vi "save_batch+info_files.vi.vi"(0 "Current PulseBlaster Array":T5(array[cluster]), 1 "6713 DAC Array":dbl[](array[numeric]), 2 "Save in second location?":bool, 3 "detuning values":T4={"flaser"=-22.0, "fimage"=14.997, "fmot"=-56.5, "fzeeman"=-524.0, "f2dcollimator"=-22.0, "fmolecule"=-2225.6} {"fmolecule" format="%.2f"; "f2dcollimator" format="%.2f"; "fzeeman" format="%.2f"; "fmot" format="%.2f"; "fimage" format="%.2f"; "flaser" format="%.2f"}, 4 "2scope filename":string, 5 "wavemeter reading":string, 6 "Drop Time Column":i32=16, 7 "Parameters to Change":T1={"PB parameter to change"=0, "Column of\nData to Change"=0, "Column of\nDelay to Change"=9, "6713 DAC Ch\nto Change"=7, "column for Wvfrm\n(red mot cooling)"=10, "# of PB arrays"=1, "column for Wvrm\nODT"=10, "TrimCurrent\nCh to Chng"=1} {"TrimCurrent\nCh to Chng" min=1 max=2; "PB parameter to change" min=0 max=4}, 8 "base path":path, 9 "saved image dimensions":i32[](array[numeric]), 10 "Cut Images\nin Software?":bool=TRUE, 11 "Array of monitor outputs":dbl[](array[numeric]), 12 "ROI Parameters":T2={"Col Start"=45, "Col Length"=125, "Row Start"=105, "Row Length"=130}, 13 "Software Binning\n(occurs before saving)":T3={"Software\nBinning?"=TRUE, "Software Bin Size"=4}, 14 "Base File Name":string="redMOTtemp0441" caption="Base File Name (filename, base delay of column 10, and .dat will be added as extension.", 15 "Changed Value":dbl=165.25000000000003, 16 "arbitrary info string":string, 17 "Software\nSumming":u32=10, 18 "alternate path":path, 19 "Analog Input Ch \nto Save to Batch":i32, 20 "Opt trap Wvfrm array":waveform(dbl)[](array[waveform]), 22 "ODT Wvfrm trigger column":i32=16, 23 "PixelFly y bin":i32, 24 "PixelFly x bin":i32, 26 "Opt Trap off column":i32=16, 27 "iteration #":i32) -> (25 "filename component":string)   [LabVIEW 2013]
doc: "This VI concatenates various information of interest to form the file name component that goes before the extension (and possibly another modifier such as \"atoms\" or \"background\")."
uses:
  <vilib>/Waveform/WDTOps.llb/WDT Index Channel DBL.vi
  <vilib>/Waveform/WDTOps.llb/WDT Waveform Duration DBL.vi
  <vilib>/Waveform/WDTOps.llb/WDT Get XY Value DBL.vi
panel:
  in  "BEC Peak weight":i32
  in  "Thermal width guess":i32=10
  in  "BEC width guess":i32=25
  out "6713 dac1 string":string
  out "6713 DAC CH0":string
  out "waveform 2":waveform(dbl)(graph)
  out "waveform":waveform(dbl)(graph)
  out "Dimple value":dbl format="%.3f"
  out "ODT value":dbl format="%.3f"
  in  "Gain (har wired)":i32(ring) items=["Low (X1)", "High (X2)"]
  out "opt trap off time (along wvfrm)":dbl
  in  "Image Beam Column":i32=23
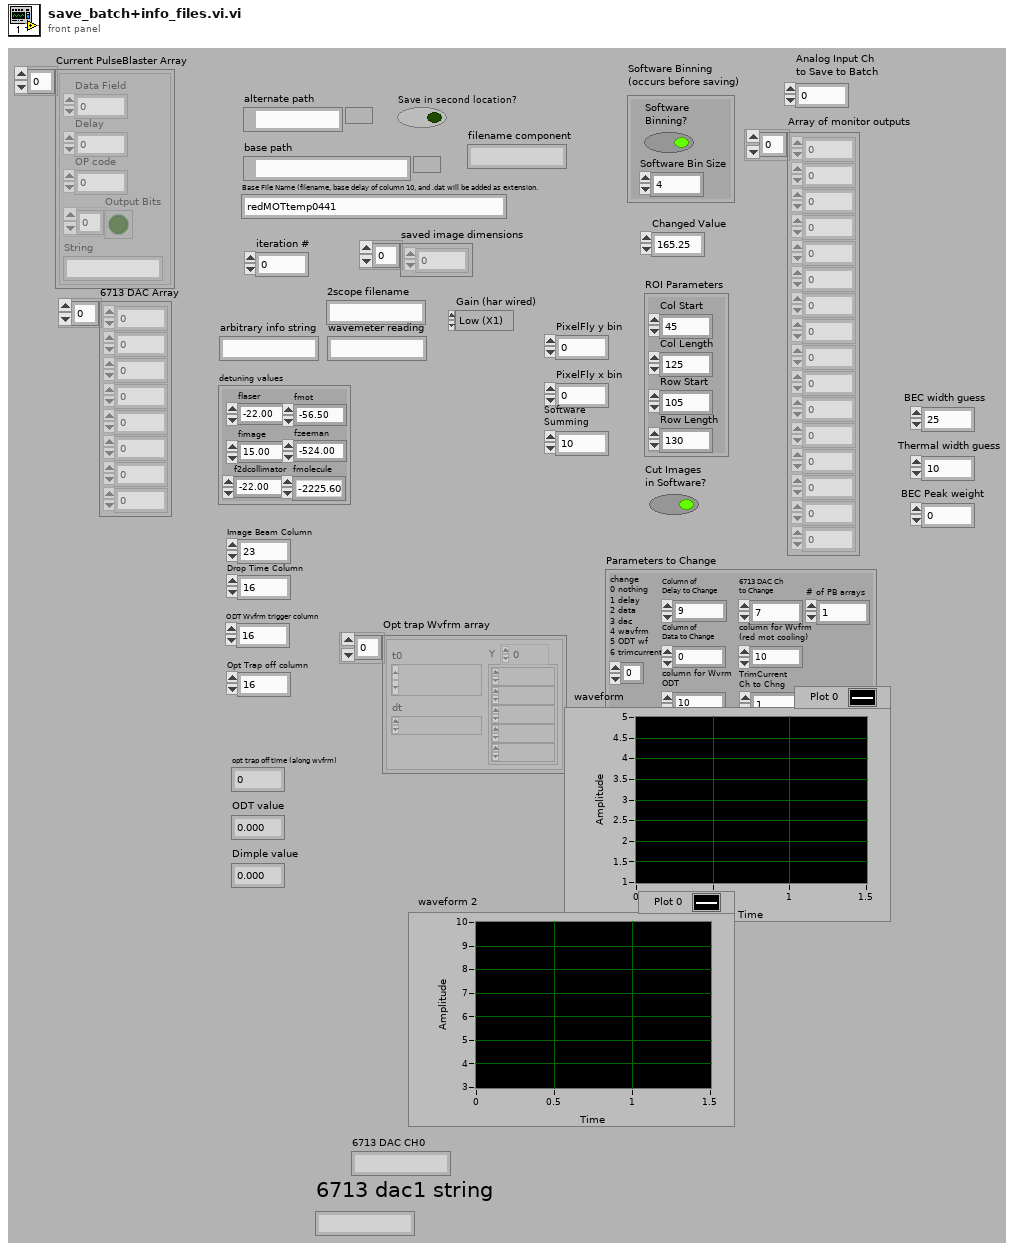
[diagram p1: front panel]
types:
  T1 = cluster{"PB parameter to change":i8, "Column of\nData to Change":i32, "Column of\nDelay to Change":i32, "6713 DAC Ch\nto Change":i32, "column for Wvfrm\n(red mot cooling)":i32, "# of PB arrays":i32, "column for Wvrm\nODT":i32, "TrimCurrent\nCh to Chng":i32}
  T2 = cluster{"Col Start":i32, "Col Length":i32, "Row Start":i32, "Row Length":i32}
  T3 = cluster{"Software\nBinning?":bool, "Software Bin Size":i32}
  T4 = cluster{"flaser":dbl, "fimage":dbl, "fmot":dbl, "fzeeman":dbl, "f2dcollimator":dbl, "fmolecule":dbl}
  T5 = cluster{"Data Field":u32, "Delay":dbl, "OP code":u8, "Output Bits":bool[], "String":string}[]
  T6 = cluster{"Data Field":u32, "Delay":dbl, "OP code":u8, "Output Bits":bool[], "String":string}
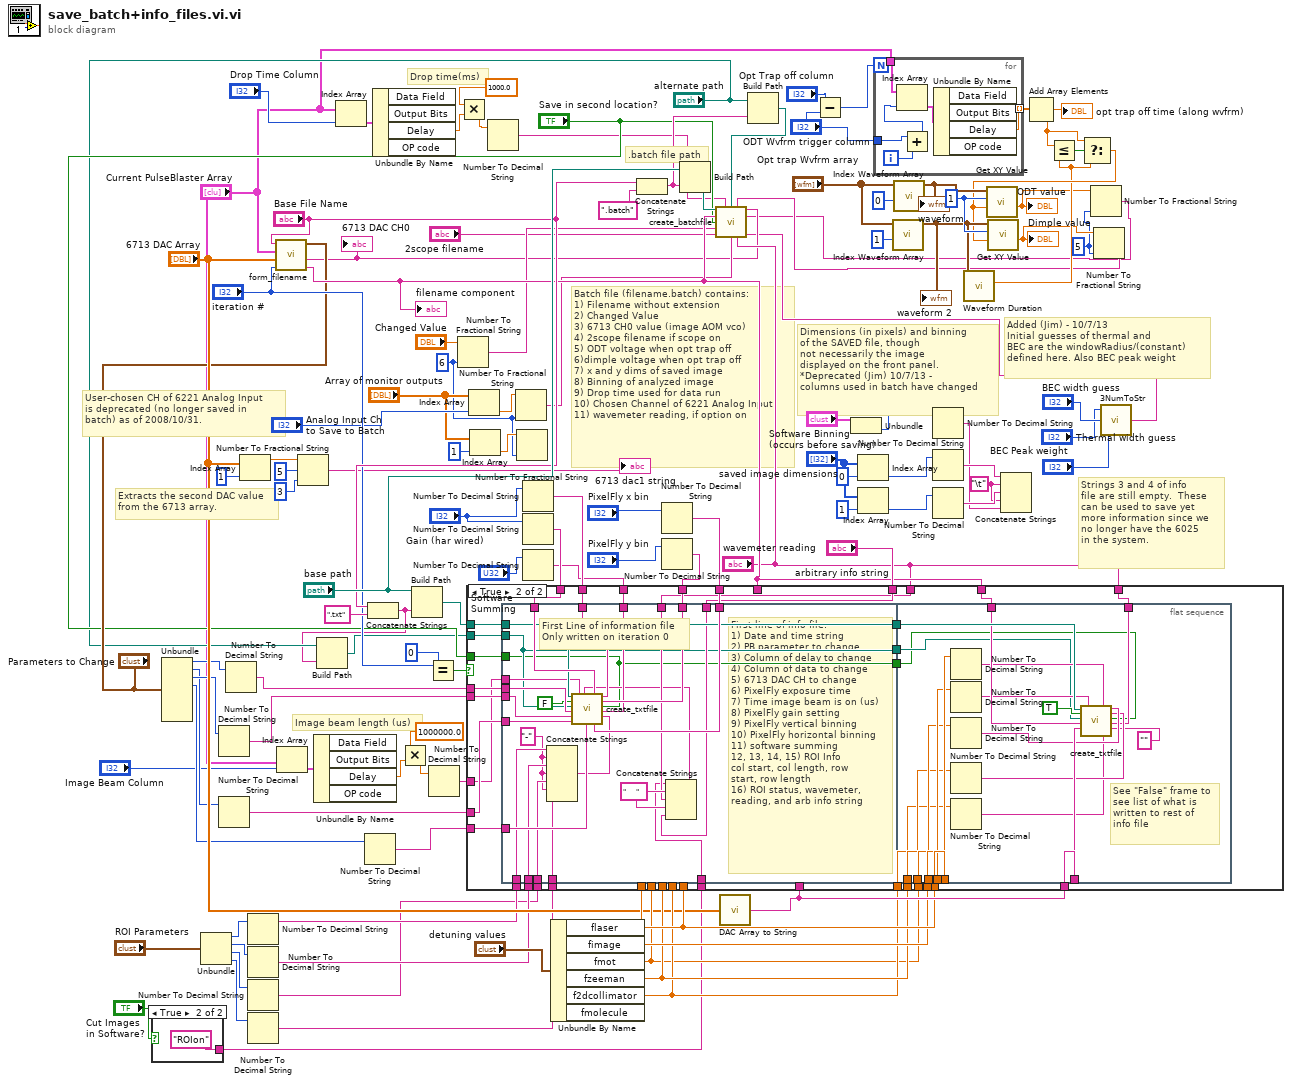
[diagram p0: block diagram]
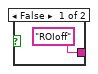
[diagram p2: hidden frame]
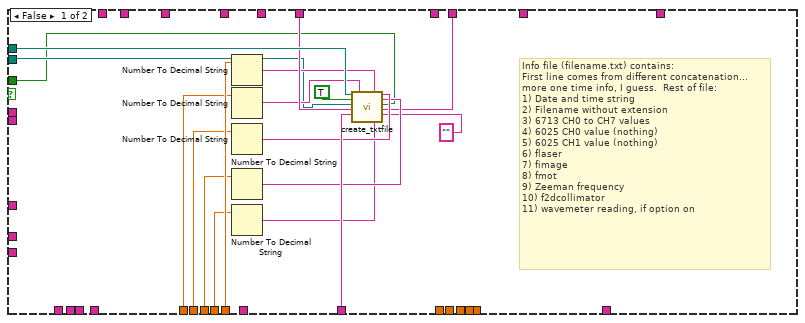
[diagram p3: hidden frame]
diagram:
  w5 = i16 5 ("width (-)")
  w18 = 1 ("index")
  w42 = i16 6 ("precision (6)")
  w61 = "\t"
  # "Added (Jim) - 10/7/13\nInitial guesses of thermal and\nBEC are the windowRadius/(constant) \ndefined here. Also BEC peak weight"
  # "User-chosen CH of 6221 Analog Input\nis deprecated (no longer saved in \nbatch) as of 2008/10/31."
  # "Drop time(ms)"
  # "Dimensions (in pixels) and binning\nof the SAVED file, though\nnot necessarily the image\ndisplayed on the front panel.\n*Deprecated (Jim) 10/7/13 - \ncolumns used in batch have changed"
  # ".batch file path"
  # "Strings 3 and 4 of info\nfile are still empty.  These\ncan be used to save yet\nmore information since we\nno longer have the 6025\nin the system."
  # "Extracts the second DAC value\nfrom the 6713 array."
  # "Image beam length (us)"
  # "Batch file (filename.batch) contains:\n1) Filename without extension\n2) Changed Value\n3) 6713 CH0 value (image AOM vco)\n4) 2scope filename if scope on\n5) ODT voltage when opt trap off\n6)dimple voltage when opt trap off\n7) x and y dims of saved image\n8) Binning of analyzed image\n9) Drop time used for data run\n10) Chosen Channel of 6221 Analog Input\n11) wavemeter reading, if option on"
  n1 = case shown="True" "Cut Images\nin Software?" {
    tunnel: ["ROIoff" "ROIon"] -> w49
    frame False {
    }
    frame True {
    }
  }
  n2 = Unbundle("Parameters to Change") -> ("PB parameter to change"=w78:i8, "Column of\nData to Change"=w76:i32, "Column of\nDelay to Change"=w77:i32, "6713 DAC Ch\nto Change"=w75:i32)  [unwired: 4 out]
  n3 = Unbundle("ROI Parameters") -> ("Col Start"=w58:i32, "Col Length"=w57:i32, "Row Start"=w56:i32, "Row Length"=w55:i32)
  n4 = Number To Decimal String(number=w77) -> (decimal integer string=w114:string)  [unwired: 1 in]
  n5 = Number To Decimal String(number=w76) -> (decimal integer string=w113:string)  [unwired: 1 in]
  n6 = Number To Decimal String(number=w78) -> (decimal integer string=w115:string)  [unwired: 1 in]
  n7 = Index Array(array="6713 DAC Array", index=1 ("Index")) -> (element=w89:dbl)
  n8 = Number To Decimal String(number=w58) -> (decimal integer string=w54:string)  [unwired: 1 in]
  n9 = Number To Decimal String(number=w57) -> (decimal integer string=w53:string)  [unwired: 1 in]
  n10 = Number To Decimal String(number=w56) -> (decimal integer string=w52:string)  [unwired: 1 in]
  n11 = Number To Decimal String(number=w55) -> (decimal integer string=w51:string)  [unwired: 1 in]
  n12 = call "form_filename.vi"("Parameters to Change"="Parameters to Change", "iteration #"="iteration #", "6713 DAC Array"="6713 DAC Array", "Current PulseBlaster Array"="Current PulseBlaster Array", "Base File Name"="Base File Name") -> ("filename component"=w79:string, "6713 DAC CH0"=w7:string)  [unwired: 1 out]
  "filename component" <- w79
  "6713 DAC CH0" <- w7
  n13 = Index Array(array="Current PulseBlaster Array", index="Image Beam Column") -> (element=w103:T6)
  n14 = Number To Fractional String(number=w89, width (-)=i16 5, precision (6)=i16 3) -> (F-format string=→"6713 dac1 string":string)  [unwired: 1 in]
  n15 = Unbundle By Name(w103) -> ("Delay"=w100:dbl)  [unwired: 3 out]
  n16 = Index Array(array="Current PulseBlaster Array", index="Drop Time Column") -> (element=w32:T6)
  n17 = Number To Decimal String(number=w75) -> (decimal integer string=w104:string)  [unwired: 1 in]
  n18 = Concatenate Strings("Base File Name", ".txt" ("Substring")) -> (w36:string)
  n19 = Build Path(base path="alternate path", name or relative path=w36) -> (appended path=w35:path)
  n20 = Unbundle By Name(w32) -> ("Delay"=w31:dbl)  [unwired: 3 out]
  n21 = Multiply(x=1000000.0, y=w100) -> (x*y=w98:dbl)
  n22 = Build Path(base path="base path", name or relative path=w36) -> (appended path=w85:path)
  n23 = Equal?(x="iteration #", y=0) -> (x = y?=w116:bool)
  n24 = Number To Decimal String(number=w98) -> (decimal integer string=w97:string)  [unwired: 1 in]
  n25 = Number To Fractional String(number="Changed Value", precision (6)=w42) -> (F-format string=w66:string)  [unwired: 2 in]
  n26 = Multiply(x=1000.0, y=w31) -> (x*y=w29:dbl)
  n27 = Index Array(array="Array of monitor outputs", index="Analog Input Ch \nto Save to Batch") -> (element=w48:dbl)
  n28 = Index Array(array="Array of monitor outputs", index=1) -> (element=w43:dbl)
  n29 = Number To Decimal String(number=w29) -> (decimal integer string=w28:string)  [unwired: 1 in]
  n30 = Number To Fractional String(number=w48, precision (6)=w42) -> (F-format string=w27:string)  [unwired: 2 in]
  n31 = Number To Fractional String(number=w43, precision (6)=w42) -> ()  [unwired: 2 in, 1 out]
  n32 = Number To Decimal String(number="Gain (har wired)") -> (decimal integer string=w108:string)  [unwired: 1 in]
  n33 = Number To Decimal String(number="Gain (har wired)") -> (decimal integer string=w109:string)  [unwired: 1 in]
  n34 = Number To Decimal String(number="Software\nSumming") -> (decimal integer string=w102:string)  [unwired: 1 in]
  n35 = Unbundle By Name("detuning values") -> ("flaser"=w96:dbl, "fimage"=w95:dbl, "fmot"=w88:dbl, "fzeeman"=w94:dbl, "f2dcollimator"=w93:dbl)  [unwired: 1 out]
  n36 = Concatenate Strings("Base File Name", ".batch" ("Substring")) -> (w40:string)
  n37 = Number To Decimal String(number="PixelFly x bin") -> (decimal integer string=w106:string)  [unwired: 1 in]
  n38 = Number To Decimal String(number="PixelFly y bin") -> (decimal integer string=w107:string)  [unwired: 1 in]
  n39 = Build Path(base path="base path", name or relative path=w40) -> (appended path=w86:path)
  n40 = call "DAC Array to String.vi"("6713 Write"="6713 DAC Array") -> ("string"=w101:string)
  n41 = case shown="True" w116 {
    tunnel: w115 -> [_ w169]
    tunnel: w114 -> [_ w168]
    tunnel: w113 -> [_ w167]
    tunnel: w109 -> [_ w166]
    tunnel: w108 -> [_ w165]
    tunnel: w107 -> [_ w164]
    tunnel: w106 -> [_ w163]
    tunnel: w85 -> [w138 w162]
    tunnel: w101 -> [w135 _]
    tunnel: w79 -> [w136 _]
    tunnel: "wavemeter reading" -> [w129 w159]
    tunnel: "arbitrary info string" -> [_ w160]
    tunnel: w104 -> [_ w158]
    tunnel: w102 -> [_ w157]
    tunnel: w79 -> [_ w156]
    tunnel: w101 -> [_ w155]
    tunnel: w97 -> [_ w154]
    tunnel: w96 -> [w128 _]
    tunnel: w95 -> [w127 _]
    tunnel: w88 -> [w126 _]
    tunnel: w94 -> [w125 _]
    tunnel: w93 -> [w124 _]
    tunnel: w96 -> [_ w153]
    tunnel: w95 -> [_ w152]
    tunnel: w88 -> [_ w151]
    tunnel: w94 -> [_ w150]
    tunnel: w93 -> [_ w149]
    tunnel: "wavemeter reading" -> [_ w148]
    tunnel: w54 -> [_ w147]
    tunnel: w53 -> [_ w146]
    tunnel: w52 -> [_ w145]
    tunnel: w51 -> [_ w144]
    tunnel: w49 -> [_ w143]
    tunnel: w35 -> [w122 w142]
    tunnel: "Save in second location?" -> [w121 w141]
    frame False {
      # "Info file (filename.txt) contains:\nFirst line comes from different concatenation...\nmore one time info, I guess.  Rest of file:\n1) Date and time string\n2) Filename without extension\n3) 6713 CH0 to CH7 values\n4) 6025 CH0 value (nothing)\n5) 6025 CH1 value (nothing)\n6) flaser\n7) fimage\n8) fmot\n9) Zeeman frequency\n10) f2dcollimator\n11) wavemeter reading, if option on"
      n42 = Number To Decimal String(number=w128) -> (decimal integer string=w134:string)  [unwired: 1 in]
      n43 = Number To Decimal String(number=w127) -> (decimal integer string=w133:string)  [unwired: 1 in]
      n44 = Number To Decimal String(number=w126) -> (decimal integer string=w132:string)  [unwired: 1 in]
      n45 = Number To Decimal String(number=w125) -> (decimal integer string=w131:string)  [unwired: 1 in]
      n46 = Number To Decimal String(number=w124) -> (decimal integer string=w130:string)  [unwired: 1 in]
      n47 = call "create_txtfile.vi"("appended path"=w138, "append to file? (new file:F)"=TRUE, "alternate path"=w122, "String"=w136, "String 2"=w135, "String 6"=w133, "String 5"=w134, "String 9"=w130, "String 7"=w132, "String 8"=w131, "Save in second location?"=w121, "String 10"=w129, "String 11"="") -> ()  [unwired: 6 in, 1 out]
    }
    frame True {
      n48 = flat-sequence {
        tunnel: w169 -> [w194]
        tunnel: w168 -> [w193]
        tunnel: w167 -> [w192]
        tunnel: w166 -> [w191]
        tunnel: w165 -> [w190]
        tunnel: w164 -> [w189]
        tunnel: w163 -> [w188]
        tunnel: w162 -> [w186]
        tunnel: [w186] -> w161
        tunnel: w160 -> [w181]
        tunnel: w159 -> [w180]
        tunnel: w158 -> [w185]
        tunnel: w157 -> [w184]
        tunnel: w154 -> [w183]
        tunnel: w147 -> [w176]
        tunnel: w146 -> [w175]
        tunnel: w145 -> [w174]
        tunnel: w144 -> [w173]
        tunnel: w143 -> [w179]
        tunnel: w142 -> [w171]
        tunnel: w141 -> [w170]
        tunnel: [w171] -> w140
        tunnel: [w170] -> w139
        tunnel: w161 -> [w211]
        tunnel: w156 -> [w210]
        tunnel: w155 -> [w209]
        tunnel: w153 -> [w208]
        tunnel: w152 -> [w207]
        tunnel: w151 -> [w206]
        tunnel: w150 -> [w205]
        tunnel: w149 -> [w204]
        tunnel: w148 -> [w197]
        tunnel: w140 -> [w196]
        tunnel: w139 -> [w195]
        frame #0 {
          w172 = "-"
          w182 = "     " ("string")
          # "First line of info file: \n1) Date and time string\n2) PB parameter to change\n3) Column of delay to change\n4) Column of data to change\n5) 6713 DAC CH to change\n6) PixelFly exposure time\n7) Time image beam is on (us)\n8) PixelFly gain setting\n9) PixelFly vertical binning\n10) PixelFly horizontal binning\n11) software summing\n12, 13, 14, 15) ROI Info\ncol start, col length, row\nstart, row length\n16) ROI status, wavemeter, \nreading, and arb info string"
          # "First Line of information file\nOnly written on iteration 0"
          n49 = Concatenate Strings(w176, w172, w175, w172, w174, w172, w173) -> (w178:string)
          n50 = Concatenate Strings(w179, w182, w180, w182, w181) -> (w177:string)
          n51 = call "create_txtfile.vi"("appended path"=w186, "append to file? (new file:F)"=FALSE, "alternate path"=w171, "String"=w194, "String 2"=w193, "String 3"=w192, "String 6"=w183, "String 4"=w185, "String 12"=w177, "String 5"=w191, "String 9"=w188, "String 7"=w190, "String 8"=w189, "Save in second location?"=w170, "String 10"=w184, "String 11"=w178) -> ()  [unwired: 3 in, 1 out]
        }
        frame #1 {
          # "See \"False\" frame to\nsee list of what is\nwritten to rest of\ninfo file"
          n52 = Number To Decimal String(number=w208) -> (decimal integer string=w203:string)  [unwired: 1 in]
          n53 = Number To Decimal String(number=w207) -> (decimal integer string=w202:string)  [unwired: 1 in]
          n54 = Number To Decimal String(number=w206) -> (decimal integer string=w201:string)  [unwired: 1 in]
          n55 = Number To Decimal String(number=w205) -> (decimal integer string=w200:string)  [unwired: 1 in]
          n56 = Number To Decimal String(number=w204) -> (decimal integer string=w199:string)  [unwired: 1 in]
          n57 = call "create_txtfile.vi"("appended path"=w211, "append to file? (new file:F)"=TRUE, "alternate path"=w196, "String"=w210, "String 2"=w209, "String 6"=w202, "String 5"=w203, "String 9"=w199, "String 7"=w201, "String 8"=w200, "Save in second location?"=w195, "String 10"=w197, "String 11"="") -> ()  [unwired: 6 in, 1 out]
        }
      }
    }
  }
  n58 = Build Path(base path="alternate path", name or relative path=w40) -> (appended path=w39:path)
  n59 = Subtract(x="Opt Trap off column", y="ODT Wvfrm trigger column") -> (x-y=w25:i32)
  n60 = Unbundle("Software Binning\n(occurs before saving)") -> ("Software Bin Size"=w62:i32)  [unwired: 1 out]
  n61 = Index Array(array="saved image dimensions", index=0) -> (element=w71:i32)
  n62 = Index Array(array="saved image dimensions", index=1) -> (element=w70:i32)
  n63 = for {
    N: w25 -> [_]
    tunnel: "Current PulseBlaster Array" -> [w217]
    tunnel: "ODT Wvfrm trigger column" -> [w215]
    tunnel: [w213] -> w17 mode=indexing
    i -> [w216]
    n64 = Add(x=w215, y=w216) -> (x+y=w214:i32)
    n65 = Index Array(array=w217, index=w214) -> (element=w218:T6)
    n66 = Unbundle By Name(w218) -> ("Delay"=w213:dbl)  [unwired: 3 out]
  }
  n67 = call-poly <vilib>:"Index Waveform Array.vi"("index"=1, "waveform array"="Opt trap Wvfrm array") -> ("waveform"=w15:waveform(dbl))  [unwired: 8 in, 1 out]
  "waveform 2" <- w15
  n68 = call-poly <vilib>:"Index Waveform Array.vi"("index"=0, "waveform array"="Opt trap Wvfrm array") -> ("waveform"=w21:waveform(dbl))  [unwired: 8 in, 1 out]
  "waveform" <- w21
  n69 = Number To Decimal String(number=w62) -> (decimal integer string=w60:string)  [unwired: 1 in]
  n70 = Number To Decimal String(number=w71) -> (decimal integer string=w69:string)  [unwired: 1 in]
  n71 = Number To Decimal String(number=w70) -> (decimal integer string=w68:string)  [unwired: 1 in]
  n72 = call-poly <vilib>:"Waveform Duration.vi"("waveform in"=w15) -> ("duration"=w11:dbl)  [unwired: 8 in, 2 out]
  n73 = Concatenate Strings(w69, w61, w68, w61, w60) -> ()  [unwired: 1 out]
  n74 = Add Array Elements(numeric array=w17) -> (sum=w13:dbl)
  "opt trap off time (along wvfrm)" <- w13
  n75 = Less Or Equal?(x=w13, y=w11) -> (x <= y?=w14:bool)
  n76 = Select(t=w13, s=w14, f=w11) -> (s? t:f=w12:dbl)
  n77 = call-poly <vilib>:"Get XY Value.vi"("Y position"=w12, "Y position format"=w18, "waveform in"=w21) -> ("Y value"=w10:dbl)  [unwired: 4 in, 4 out]
  "ODT value" <- w10
  n78 = call-poly <vilib>:"Get XY Value.vi"("Y position"=w12, "Y position format"=w18, "waveform in"=w15) -> ("Y value"=w9:dbl)  [unwired: 4 in, 4 out]
  "Dimple value" <- w9
  n79 = Number To Fractional String(number=w10, precision (6)=w5) -> (F-format string=w6:string)  [unwired: 2 in]
  n80 = Number To Fractional String(number=w9, precision (6)=w5) -> (F-format string=w8:string)  [unwired: 2 in]
  n81 = call "3NumToStr.vi"("Num 3"="BEC Peak weight", "Num 2"="BEC width guess", "Num 1"="Thermal width guess") -> ("Combined Output String"=w4:string)
  n82 = call "create_batchfile.vi"("appended path"=w86, "String 8"=w28, "alternate path"=w39, "String 6"=w8, "String 4"=w7, "String"=w79, "String 5"=w6, "Save in second location?"="Save in second location?", "String 2"=w66, "String 3"="2scope filename", "String 9"=w27, "String 10"="wavemeter reading", "String 7"=w4) -> ()  [unwired: 3 in]
